vi "MainV2.vi"() -> ()   [LabVIEW 2019]
uses:
  <vilib>/userDefined/High Color/IMAQdx.ctl
  <vilib>/Platform/TimedLoop/XDataNode/timing_clust.ctl
  <vilib>/Platform/TimedLoop/XDataNode/nitl_modes.ctl
  <vilib>/Platform/TimedLoop/XDataNode/wakeup.ctl
  <vilib>/myRIO/Instrument Drivers/Onboard IO/AO/typedefs/AO Reference.ctl
  <vilib>/myRIO/Common/Instrument Driver Framework/Utilities/typedefs/myRIO Generic Hardware Reference.ctl
  <vilib>/myRIO/Common/Instrument Driver Framework/Utilities/typedefs/Hardware Version Enum.ctl
  <vilib>/myRIO/Common/Instrument Driver Framework/Utilities/typedefs/myRIO v1.0 Reference.ctl
  <vilib>/myRIO/Common/Instrument Driver Framework/Utilities/typedefs/Generic FPGA Reference.ctl
  <vilib>/myRIO/Common/Instrument Driver Framework/myRIO v1.0/AO/typedefs/AO Channels List.ctl
  <vilib>/myRIO/Common/Instrument Driver Framework/myRIO v1.0/AO/typedefs/AO Channels Enum.ctl
  <vilib>/myRIO/Common/Instrument Driver Framework/Utilities/typedefs/Analog Scaling Constants List.ctl
  <vilib>/myRIO/Common/Instrument Driver Framework/Utilities/typedefs/Analog Scaling Constants.ctl
  <vilib>/userDefined/High Color/nirio_resource_hc.ctl
  <vilib>/myRIO/Common/Instrument Driver Framework/myRIO v1.0/Encoder/typedefs/Encoder Signal Mode.ctl
  <vilib>/myRIO/Instrument Drivers/Onboard IO/Encoder/typedefs/Encoder Reference.ctl
  <vilib>/myRIO/Common/Instrument Driver Framework/myRIO v1.0/Encoder/typedefs/Encoder Channels Enum.ctl
  <vilib>/myRIO/Common/Instrument Driver Framework/myRIO v1.0/Encoder/typedefs/Encoder Configuration v1.0.ctl
  <vilib>/myRIO/Common/Instrument Driver Framework/Utilities/vis/Is FPGA Ref Available.vi
  <vilib>/myRIO/Common/Instrument Driver Framework/myRIO v1.0/AO/vis/myRIO v1.1 Open AO.vi
  <vilib>/myRIO/Instrument Drivers/Onboard IO/AO/vis/Write.vi
  <vilib>/myRIO/Common/Instrument Driver Framework/myRIO v1.0/Encoder/vis/myRIO v1.1 Open Encoder.vi
  <vilib>/myRIO/Instrument Drivers/Onboard IO/Encoder/vis/Read.vi
  <vilib>/myRIO/Common/Instrument Driver Framework/Utilities/vis/Validate Channels.vi
  <vilib>/myRIO/Common/Instrument Driver Framework/myRIO v1.0/AO/vis/myRIO v1.0 Reserve AO.vi
  <vilib>/myRIO/Common/Instrument Driver Framework/myRIO v1.0/Encoder/vis/myRIO v1.0 Reserve Encoder.vi
  <vilib>/myRIO/Common/Instrument Driver Framework/myRIO v1.0/AO/vis/myRIO v1.0 Build MUX Configuration AO.vi
  <vilib>/myRIO/Common/Instrument Driver Framework/myRIO v1.0/Resource Manager/vis/myRIO v1.0 Reserve Channel List.vi
  <vilib>/myRIO/Common/Instrument Driver Framework/myRIO v1.0/Encoder/vis/myRIO v1.0 Build MUX Configuration Encoder.vi
  <vilib>/myRIO/Common/Instrument Driver Framework/myRIO v1.0/Resource Manager/vis/myRIO v1.0 Reserve Channel.vi
  <vilib>/myRIO/Common/Instrument Driver Framework/myRIO v1.0/Resource Manager/vis/myRIO v1.0 Unreserve Channel.vi
  <vilib>/myRIO/Common/Instrument Driver Framework/myRIO v1.0/Resource Manager/vis/myRIO v1.0 Create Configuration List.vi
  <vilib>/myRIO/Common/Instrument Driver Framework/myRIO v1.0/Resource Manager/vis/myRIO v1.0 Build Mutex Name.vi
  <vilib>/Utility/VariantDataType/GetNumericInfo.vi
  <vilib>/Utility/error.llb/Error Cluster From Error Code.vi
  <vilib>/myRIO/Common/Instrument Driver Framework/myRIO v1.0/myRIO v1.1 Open.vi
  <vilib>/myRIO/Common/Instrument Driver Framework/myRIO v1.0/AO/vis/myRIO v1.0 Get Scaling Constants AO.vi
  <vilib>/myRIO/Common/Instrument Driver Framework/Utilities/vis/IO Manager.vi
  <vilib>/myRIO/Common/Instrument Driver Framework/Utilities/vis/Configuration Manager.vi
  <vilib>/myRIO/Common/Instrument Driver Framework/myRIO v1.0/myRIO v1.0 Close.vi
  <vilib>/myRIO/Common/Instrument Driver Framework/myRIO v1.0/AO/vis/myRIO v1.0 Write AO.vi
  <vilib>/myRIO/Common/Instrument Driver Framework/myRIO v1.0/Resource Manager/vis/myRIO v1.0 Configure IO.vi
  <vilib>/myRIO/Common/Instrument Driver Framework/myRIO v1.0/Encoder/vis/myRIO v1.0 Configure Encoder.vi
  <vilib>/myRIO/Common/Instrument Driver Framework/myRIO v1.0/Encoder/vis/myRIO v1.0 Read Encoder.vi
  <vilib>/platform/TimedLoop/XDataNode/XDataNode.xnode
  <vilib>/myRIO/Express VI/Onboard IO/AO/AO Express VI.xnode
  <vilib>/myRIO/Instrument Drivers/Onboard IO/AO/vis/myRIO AO Open.xnode
  <vilib>/myRIO/Express VI/Onboard IO/Encoder/Encoder Express VI.xnode
  <vilib>/myRIO/Instrument Drivers/Onboard IO/Encoder/vis/myRIO Encoder Open.xnode
  <vilib>/myRIO/Common/Instrument Driver Framework/myRIO v1.0/Encoder/typedefs/Encoder Count Direction Enum.ctl
  <vilib>/Platform/TimedLoop/XDataNode/XDNodeRunTimeDep.lvlib
  <vilib>/myRIO/Instrument Drivers/Onboard IO/AO/AO.lvlib
  <vilib>/vision/driver/NI_Vision_Acquisition_Software.lvlib
  <vilib>/myRIO/Instrument Drivers/Onboard IO/Encoder/Encoder.lvlib
  <vilib>/vision/NI_Vision_Development_Module.lvlib
panel:
  out "error out":errorcluster
  out "appended path":path
  in  "base path":path
  in  "record_name":string
  in  "start_recording":bool
  out "record_t":dbl[](array[numeric])
  out "target_angle_y_a_target":dbl(knob) scale=-45.0..45.0
  out "target_angle_x_a_target":dbl(knob) scale=-45.0..45.0
  in  "p_ki":dbl
  in  "p_kd":dbl
  in  "p_kp":dbl
  out "y_angle":dbl(knob) scale=-45.0..45.0
  out "x_angle":dbl(knob) scale=-45.0..45.0
  out "y_error":dbl
  out "x_error":dbl
  in  "y_target":dbl(slide) scale=-1.0..1.0
  in  "x_target":dbl(slide) scale=-1.0..1.0
  out "y":dbl
  out "x":dbl
  in  "threshold":cluster{"Lower value":sgl, "Upper value":sgl}={"Lower value"=128.0, "Upper value"=255.0} {"Upper value" format="%.2f"; "Lower value" format="%.2f"}
  in  "Optional Rectangle":i32[](array[numeric])
  out "threshold":T1(plugin-control)
  out "x-y":u32
  out "y_input":dbl
  in  "a_ki":dbl
  out "y_angle_error":dbl
  in  "a_kd":dbl
  in  "a_kp":dbl
  out "x_angle_error":dbl
  in  "stop":bool
  out "x_input":dbl
  in  "reset":bool
  in  "dt":dbl
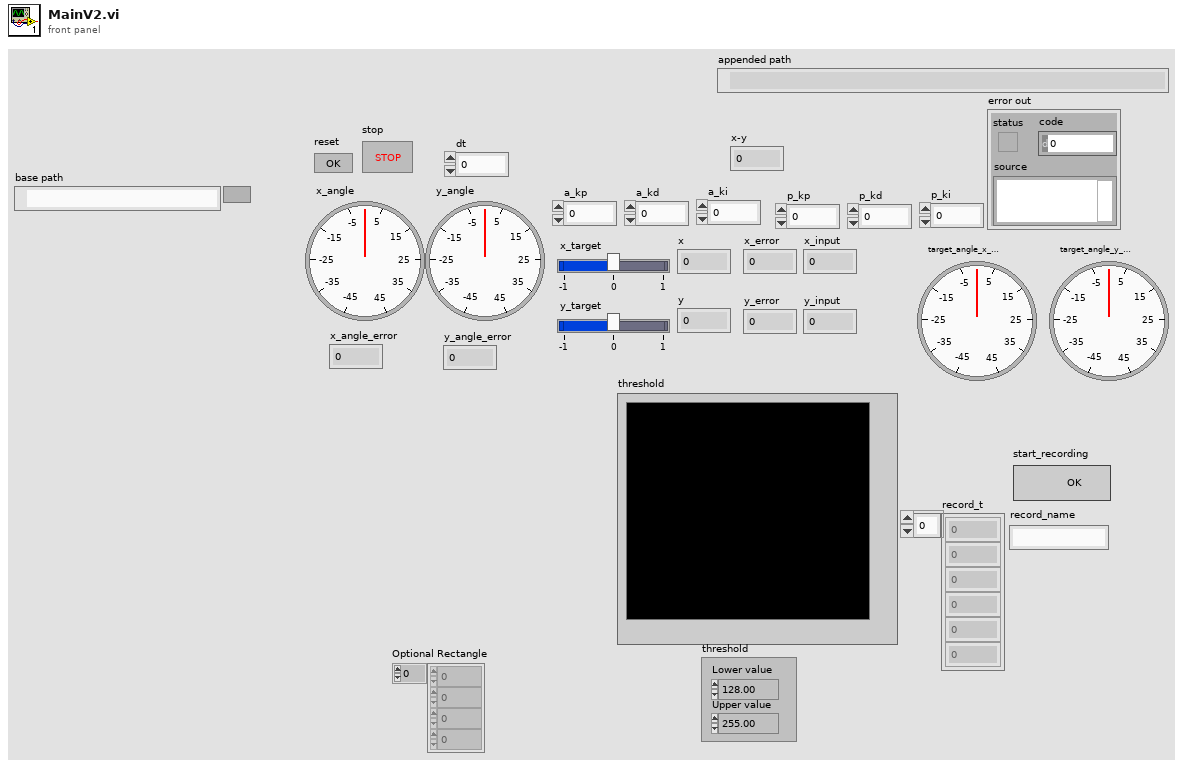
[diagram p1: front panel]
types:
  T1 = typedef "IMAQ Image.ctl" = refnum<image>
  T2 = typedef "IMAQdx.ctl" = refnum<k21>
  T3 = typedef "XDNodeRunTimeDep.lvlib/timing_clust.ctl" = cluster{"Expected End [f-1]":u64, "Actual End [f-1]":u64, "Finished Late? [f-1]":bool, "Expected End [i-1]":u64, "Actual End [i-1]":u64, "Finished Late? [i-1]":bool, "Expected Start [i]":u64, "Actual Start [i]":u64, "Expected Start [f]":u64, "Actual Start [f]":u64, "Source Name":string, "Structure Name":string, "Period":i64, "Deadline":i64, "Offset":i64, "Start":i64, "Priority":i32, "Timeout":i32, "Mode":T4, "Wakeup Reason":T5, "Error":errorcluster, "Source Type":string, "Secondary Source Type":string, "Global End Time":u64, "Global Start Time":u64, "Frame Duration":u64, "Iteration Duration":u64, "Assigned CPU":i32, "I/O Scan Engine Mode":u32}
  T4 = typedef "XDNodeRunTimeDep.lvlib/nitl_modes.ctl" = enum32{"No Change", "Process missed periods, maintain original phase", "Discard missed periods, maintain original phase", "Process missed periods, ignore original phase", "Discard missed periods, ignore original phase"}
  T5 = typedef "XDNodeRunTimeDep.lvlib/wakeup.ctl" = enum32{"Normal", "Aborted", "Asynchronous wakeup", "Timing source error", "Timed loop error", "Timeout"}
  T6 = typedef "Encoder.lvlib/Encoder Reference.ctl" = cluster{"myRIO Reference":T7, "Encoder Channels Enum":T11}
  T7 = typedef "myRIO Generic Hardware Reference.ctl" = cluster{"myRIO Model":T8, "myRIO Hardware Reference":T9}
  T8 = typedef "Hardware Version Enum.ctl" = enum16{"Unknown", "myRIO-1900", "myRIO-1950", "roboRIO", "NI ELVIS RIO CM", "ELVIS III"}
  T9 = typedef "myRIO v1.0 Reference.ctl" = cluster{"Generic FPGA Reference":T10, "Allow multiple opens":bool}
  T10 = typedef "Generic FPGA Reference.ctl" = refnum<k20>
  T11 = typedef "Encoder Channels Enum.ctl" = enum16{"Not Connected", "C/ENC0", "C/ENC1", "A/ENC", "A/ENC0", "A/ENC1", "A/ENC2", "A/ENC3", "A/ENC4", "A/ENC5", "A/ENC6", "A/ENC7", "A/ENC8", "A/ENC9", "B/ENC", "B/ENC0", "B/ENC1", "B/ENC2", "B/ENC3", "B/ENC4", "B/ENC5", "B/ENC6", "B/ENC7", "B/ENC8", "B/ENC9", "DIO/ENC0", "DIO/ENC1", "DIO/ENC2", "DIO/ENC3", "DIO/ENC4"}
  T12 = typedef "Encoder Signal Mode.ctl" = enum16{"Quadrature phase signal", "Step and direction signal"}
  T13 = typedef "nirio_resource_hc.ctl" = tag
  T14 = typedef "AO.lvlib/AO Reference.ctl" = cluster{"myRIO Reference":T7, "AO Channel List":T15, "AO Scaling Constant List":T17}
  T15 = typedef "AO Channels List.ctl" = T16[]
  T16 = typedef "AO Channels Enum.ctl" = enum16{"Not Connected", "AudioOut/Left", "AudioOut/Right", "C/AO0", "C/AO1", "A/AO0", "A/AO1", "B/AO0", "B/AO1"}
  T17 = typedef "Analog Scaling Constants List.ctl" = T18[]
  T18 = typedef "Analog Scaling Constants.ctl" = cluster{"LSB Weight (Volts)":dbl, "Offset (Volts)":dbl, "Signed?":bool}
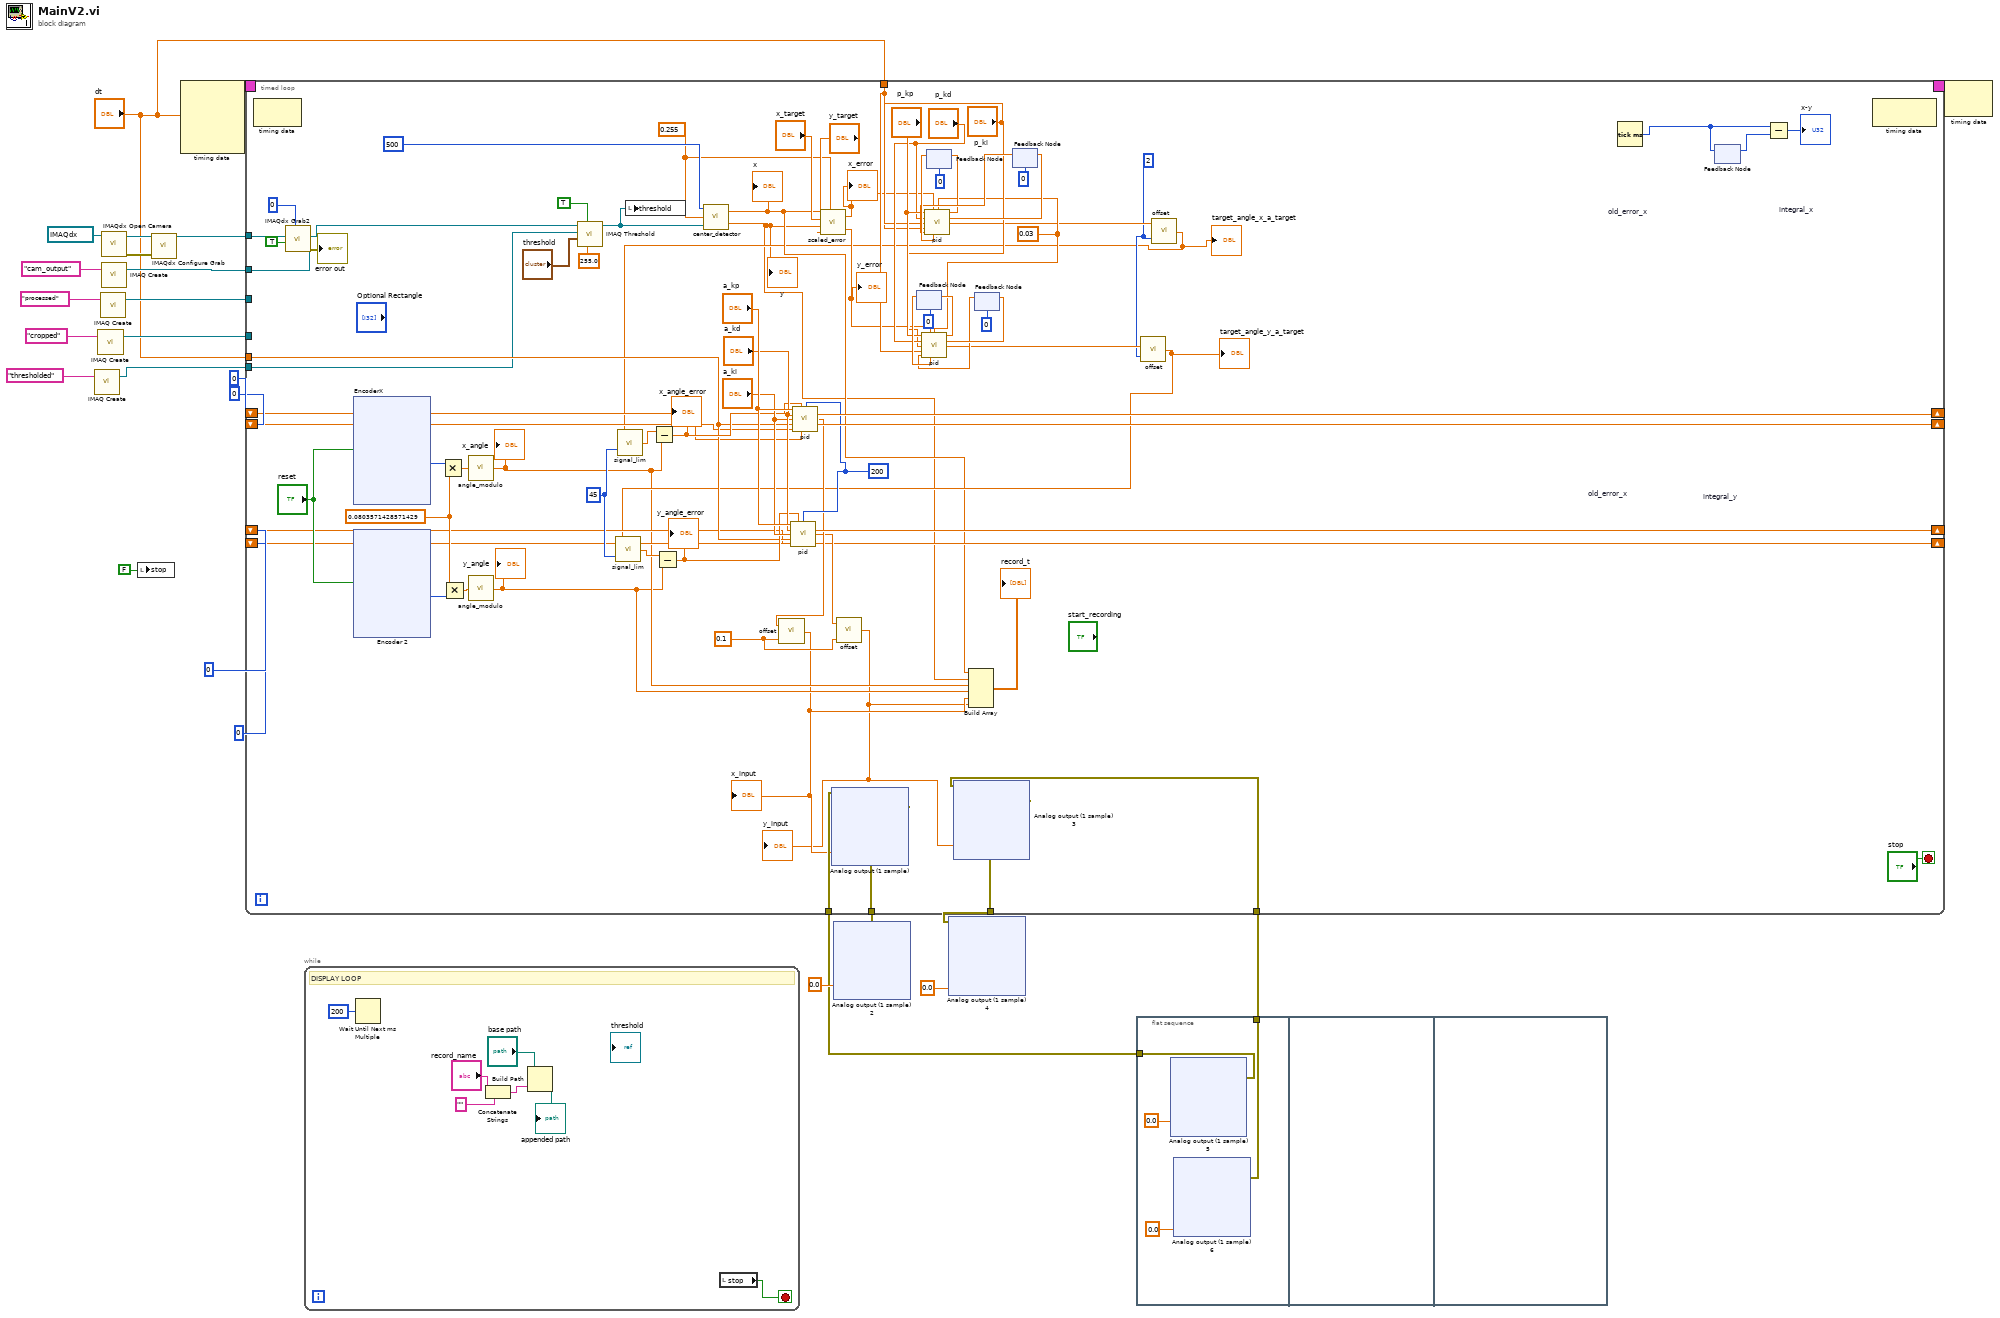
[diagram p0: block diagram]
diagram:
  n1 = call "IMAQ Create"("Image Name"="thresholded") -> ("New Image"=w3:T1)  [unwired: 4 in, 1 out]
  n2 = call "IMAQ Create"("Image Name"="cropped") -> ("New Image"=w5:T1)  [unwired: 4 in, 1 out]
  n3 = call "IMAQ Create"("Image Name"="processed") -> ("New Image"=w15:T1)  [unwired: 4 in, 1 out]
  n4 = call <vilib>:"IMAQdx Open Camera.vi"("Session In"=T2 "cam1") -> ("error out"=w18:errorcluster, "Session Out"=w19:T2)  [unwired: 9 in]
  n5 = call "IMAQ Create"("Image Name"="cam_output") -> ("New Image"=w20:T1)  [unwired: 4 in, 1 out]
  n6 = local write "stop"(FALSE ("stop")) -> ()
  n7 = call <vilib>:"IMAQdx Configure Grab.vi"("error in"=w18, "Session In"=w19) -> ("Session Out"=w21:T2)  [unwired: 8 in, 1 out]
  n8 = node-c288("dt") -> (w26:T3)  [unwired: 3 in]
  n9 = timed-loop {
    timing: w26 -> [_]
    timing-out: [_] -> w25
    tunnel: w21 -> [w107]
    tunnel: w20 -> [w106]
    tunnel: w15 -> [_]
    shift-right: [w84] -> _
    shift-left: 0 -> [w89]
    shift-right: [w83] -> _
    shift-left: 0 -> [w88]
    shift-right: [w40] -> _
    shift-left: 0 -> [w87]
    shift-right: [w85] -> _
    shift-left: 0 -> [w86]
    tunnel: "dt" -> [w90]
    tunnel: [w82] -> w10
    tunnel: [w78] -> w9
    tunnel: w8 -> [w77]
    tunnel: w7 -> [w76]
    tunnel: w5 -> [_]
    tunnel: w3 -> [w75]
    tunnel: "dt" -> [w53]
    stop <- "stop" stop-if-true
    w41 = 2
    w47 = 0.1
    w49 = 200
    w50 = 0.03
    w48 = 0.255
    w96 = 45
    w104 = 0.0803571428571429
    n10 = node-c288() -> ()  [unwired: 1 in, 1 out]
    n11 = call <vilib>:"IMAQdx Grab2.vi"("Timeout (ms)"=0, "Wait for Next Buffer? (Yes)"=TRUE, "Image In"=w106, "Session In"=w107) -> ("error out"=→"error out":errorcluster, "Image Out"=w30:T1)  [unwired: 4 in, 2 out]
    n12 = xnode "EncoderX"("Reset Counter"="reset") -> ("Counter Value"=w105:i32)  [unwired: 1 in, 3 out]
    n13 = xnode "Encoder 2"("Reset Counter"="reset") -> ("Counter Value"=w103:i32)  [unwired: 1 in, 3 out]
    n14 = Multiply(x=w105, y=w104) -> (x*y=w100:dbl)
    n15 = Multiply(x=w104, y=w103) -> (x*y=w99:dbl)
    n16 = call "angle_modulo.vi"("alpha"=w100) -> ("alpha_prime"=w37:dbl)
    "x_angle" <- w37
    n17 = call "angle_modulo.vi"("alpha"=w99) -> ("alpha_prime"=w36:dbl)
    "y_angle" <- w36
    n18 = call "IMAQ Threshold"("Replace Value"=sgl 255.0, "Keep/Replace Value (Replace)"=TRUE, "Range"="threshold", "Image Dst"=w75, "Image Src"=w30) -> ("Image Dst Out"=w31:T1)  [unwired: 5 in, 1 out]
    n19 = local write "threshold"(w31) -> ()
    n20 = call "center_detector.vi"("Image"=w31, "size_m"=w48, "size_px"=500 ("Y Resolution")) -> ("y"=w33:dbl, "x"=w39:dbl)
    "x" <- w39
    "y" <- w33
    n21 = call "scaled_error.vi"("x"=w39, "x_target"="x_target", "y"=w33, "y_target"="y_target", "size_m"=w48) -> ("err_x"=w52:dbl, "err_y"=w51:dbl)
    "x_error" <- w52
    "y_error" <- w51
    n22 = feedback #1 "old_error_x"(0) -> (w59:dbl)
    n23 = feedback #2 "old_error_x"(0) -> (w64:dbl)
    n24 = feedback #3 "integral_y"(0) -> (w57:dbl)
    n25 = call "pid.vi"("kp"="p_kp", "err"=w51, "lim"=w50, "kd"="p_kd", "ki"="p_ki", "dt"=w53, "intergral"=w57, "old_err"=w59) -> ("curr_err"=w60:dbl, "curr_integral"=w58:dbl, "y"=w43:dbl)  [unwired: 5 in]
    n26 = feedback-in #1(w60) -> ()
    n27 = feedback-in #3(w58) -> ()
    n28 = feedback #4 "integral_x"(0) -> (w62:dbl)
    n29 = call "pid.vi"("kp"="p_kp", "err"=w52, "lim"=w50, "kd"="p_kd", "ki"="p_ki", "dt"=w53, "intergral"=w62, "old_err"=w64) -> ("curr_err"=w61:dbl, "curr_integral"=w63:dbl, "y"=w44:dbl)  [unwired: 5 in]
    n30 = feedback-in #2(w61) -> ()
    n31 = feedback-in #4(w63) -> ()
    n32 = call "offset.vi"("offset"=w41, "x"=w43) -> ("y"=w42:dbl)
    "target_angle_y_a_target" <- w42
    n33 = call "signal_lim.vi"("lim"=w96, "x"=w42) -> ("y"=w97:dbl)
    n34 = Subtract(x=w97, y=w36) -> (x-y=w91:dbl)
    "y_angle_error" <- w91
    n35 = call "pid.vi"("kp"="a_kp", "err"=w91, "lim"=w49, "kd"="a_kd", "ki"="a_ki", "dt"=w90, "intergral"=w86, "old_err"=w87) -> ("curr_err"=w40:dbl, "curr_integral"=w85:dbl, "y"=w45:dbl)  [unwired: 5 in]
    n36 = call "offset.vi"("offset"=w47, "x"=w45) -> ("y"=w34:dbl)
    "y_input" <- w34
    n37 = xnode "Analog output (1 sample) 3"("C/AO1 (AO1)"=w34, "error in (no error)"=w76) -> ("error out"=w78:errorcluster)
    n38 = call "offset.vi"("offset"=w41, "x"=w44) -> ("y"=w38:dbl)
    "target_angle_x_a_target" <- w38
    n39 = call "signal_lim.vi"("lim"=w96, "x"=w38) -> ("y"=w98:dbl)
    n40 = Subtract(x=w98, y=w37) -> (x-y=w92:dbl)
    "x_angle_error" <- w92
    n41 = call "pid.vi"("kp"="a_kp", "err"=w92, "lim"=w49, "kd"="a_kd", "ki"="a_ki", "dt"=w90, "intergral"=w88, "old_err"=w89) -> ("curr_err"=w84:dbl, "curr_integral"=w83:dbl, "y"=w46:dbl)  [unwired: 5 in]
    n42 = call "offset.vi"("offset"=w47, "x"=w46) -> ("y"=w35:dbl)
    "x_input" <- w35
    n43 = xnode "Analog output (1 sample)"("C/AO0 (AO0)"=w35, "error in (no error)"=w77) -> ("error out"=w82:errorcluster)
    n44 = Build Array(w39, w33, w37, w36, w35, w34) -> (→"record_t":dbl[])
    n45 = Tick Count (ms)() -> (millisecond timer value=w81:u32)
    n46 = feedback-in #5(w81) -> ()
    n47 = feedback #5() -> (w80:u32)  [unwired: 1 in]
    n48 = Subtract(x=w81, y=w80) -> (x-y=→"x-y":u32)
    n49 = node-c288() -> ()  [unwired: 1 in, 1 out]
  }
  n50 = while {
    stop <- w281 stop-if-true
    # "DISPLAY LOOP"
    n51 = Wait Until Next ms Multiple(millisecond multiple=u32 200) -> ()  [unwired: 1 out]
    n52 = Concatenate Strings("record_name", "") -> (w278:string)
    n53 = Build Path(base path="base path", name or relative path=w278) -> (appended path=→"appended path":path)
    n54 = local read "stop"() -> (w281:bool)
  }
  n55 = xnode "Analog output (1 sample) 2"("C/AO0 (AO0)"=0.0, "error in (no error)"=w10) -> ()  [unwired: 1 out]
  n56 = xnode "Analog output (1 sample) 4"("C/AO1 (AO1)"=0.0, "error in (no error)"=w9) -> ()  [unwired: 1 out]
  n57 = flat-sequence {
    tunnel: [w284] -> w8
    tunnel: [w283] -> w7
    frame #0 {
      n58 = xnode "Analog output (1 sample) 5"("C/AO0 (AO0)"=0.0) -> ("error out"=w284:errorcluster)  [unwired: 1 in]
      n59 = xnode "Analog output (1 sample) 6"("C/AO1 (AO1)"=0.0) -> ("error out"=w283:errorcluster)  [unwired: 1 in]
    }
    frame #1 {
    }
    frame #2 {
    }
  }
  n60 = node-c288(w25) -> ()  [unwired: 1 out]
